vi "Destroy.vi"(8 "ErrorIn":errorcluster caption="Error In(no Error)", 11 "Reference in":refnum<class "ErrorDefinitionSQLite.lvclass"> caption="Reference In") -> (0 "ErrorOut":errorcluster caption="Error Out", 3 "Reference out":refnum<class "ErrorDefinitionSQLite.lvclass"> caption="Reference Out")   [LabVIEW 2018, in "ErrorDefinitionSQLite.lvclass"]
uses:
  ErrorDefinitionSQLite.lvclass
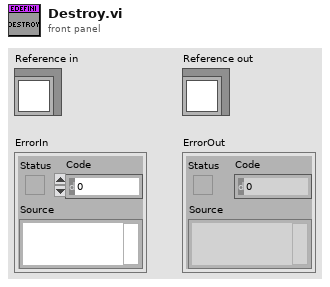
[diagram p1: front panel]
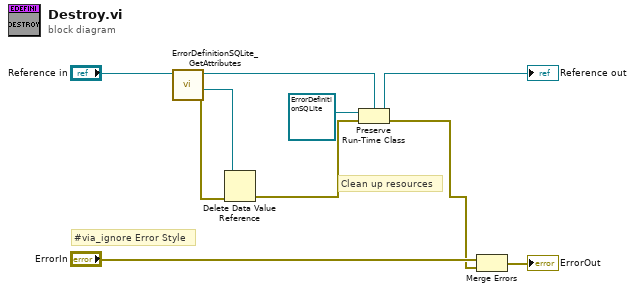
[diagram p0: block diagram]
diagram:
  # "#via_ignore Error Style"
  # "Clean up resources"
  n1 = call "ErrorDefinitionSQLite_GetAttributes.vi"("Reference in"="Reference in") -> ("ErrorOut"=w8:errorcluster, "DataRef"=w7:refnum<data-value>, "Reference out"=w4:refnum<class "ErrorDefinitionSQLite.lvclass">)  [unwired: 7 in, 1 out]
  n2 = Delete Data Value Reference(data value reference=w7, error in=w8) -> (error out=w2:errorcluster)  [unwired: 1 out]
  n3 = Preserve Run-Time Class(object in=refnum<class "ErrorDefinitionSQLite.lvclass"> refnum ("Reference out"), error in=w2, 2:w4) -> (object out=→"Reference out":refnum<class "ErrorDefinitionSQLite.lvclass">, error out=w1:errorcluster)
  n4 = Merge Errors("ErrorIn", w1) -> (→"ErrorOut":errorcluster)
